vi "08.Evd.4_Ask.1.vi"() -> ()   [LabVIEW 2020]
panel:
  in  "Delay Time (s)":dbl=1.0
  in  "stop":bool
  in  "Θερμοκρασία σε C":bool
  out "Θερμοκρασία":dbl(slide) scale=0.0..200.0
  # "Κλίμακα θερμοκρασίας"
  # "Θερμοκρασία σε F"
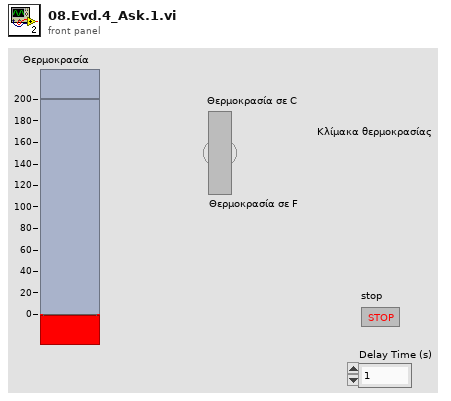
[diagram p1: front panel]
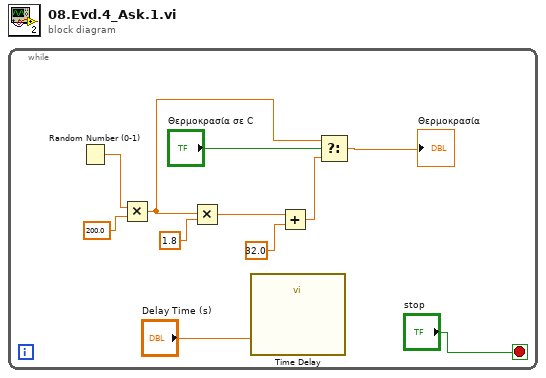
[diagram p0: block diagram]
diagram:
  n1 = while {
    stop <- "stop" stop-if-true
    n2 = Random Number (0-1)() -> (number: 0 to 1=w4:dbl)
    n3 = Multiply(x=w4, y=200.0) -> (x*y=w3:dbl)
    n4 = Multiply(x=w3, y=1.8) -> (x*y=w9:dbl)
    n5 = call "Time Delay"("Delay Time (s)"="Delay Time (s)") -> ()  [unwired: 10 in, 1 out]
    n6 = Add(x=w9, y=32.0) -> (x+y=w7:dbl)
    n7 = Select(t=w3, s="Θερμοκρασία σε C", f=w7) -> (s? t:f=→"Θερμοκρασία":dbl)
  }
